vi "MethodGuide.vi"(1 "Attributes":string[](array[string])) -> (15 "Preview":string, 16 "Canceled":bool)   [LabVIEW 2020, in "DQMHModuleNode.lvclass"]
uses:
  <resource>/Framework/Providers/Open_GDS/UML/DQMHModuleNode_class/DQMHModuleNode.lvclass
  <resource>/Framework/Providers/Open_GDS/UML/DQMHModuleNode_class/EventType.ctl
  <resource>/Framework/Providers/Open_GDS/UML/ContextHelp/ContextHelp_HelpTexts.ctl
panel:
  in  "Roundtrip : Broadcast":string caption="Name of Roundtrip Broadcast"
  in  "Type":T1
  in  "Help":bool
  in  "Cancel":bool
  in  "OK":bool
  in  "Event Name":string(combo) caption="Name of Roundtrip Request"
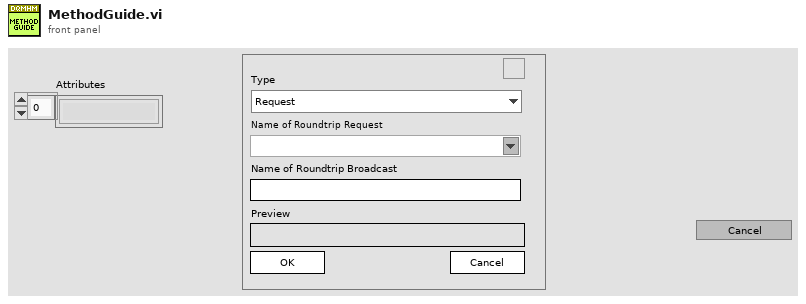
[diagram p1: front panel]
types:
  T1 = typedef "DQMHModuleNode.lvclass/EventType.ctl" = enum16{"Request", "Request and Wait For Reply", "Roundtrip", "Broadcast"}
  T2 = enum8{"Enabled", "Disabled", "Disabled and Grayed Out"}
  T3 = typedef "ContextHelp_HelpTexts.ctl" = enum16{"None(Hide)", "Default", "Help", "Welcome", "GettingStarted", "ClassDiagram_Help", "SequenceDiagram_Help", "UseCaseDiagram_Help", "BSelect", "BClass", "BInterface", "BPackage", "BNote", "BDependency", "BInheritance", "BInterfaceImplementation", "BAssociation", "BAggregation", "BCompAggregation", "BNoteConnector", "BObject", "BActionBar", "BCall", "BSystem", "BActor", "BUseCase", "BGeneralization", "BIncludes", "BExtends", "BUseCaseDiagramAssociation", "ClassRelationshipEdge editDialog_Bent Style", "ClassRelationshipEdge editDialog_RelationType", "ClassRelationshipEdge editDialog_Reverse association", "ClassRelationshipEdge editDialog_Start label", "ClassRelationshipEdge editDialog_Middle label", "ClassRelationshipEdge editDialog_End label", "UMLEditor reversedEngineering_Pathes", "ReversedEngineering StateReverseDialog_Help", "ReversedEngineering StateQueuedSettings_Help", "UMLEditor reversedEngineering_AddTopVIs", "UMLEditor reversedEngineering_AddClasses", "UMLEditor reversedEngineering_AddDirs", "UMLEditor reversedEngineering_Recursively", "UMLEditor reversedEngineering_Remove", "UMLEditor reversedEngineering_ClearList", "UMLEditor reversedEngineering_HideSubAss", "UMLEditor reversedEngineering_CreateTypes", "UMLEditor reversedEngineering_OnlyInheritance", "UMLEditor reversedEngineering_CreateApplication", "UMLEditor reversedEngineering_OK", "UMLEditor reversedEngineering_Cancel", "UMLEditor reversedEngineering_Help", "UMLEditor createWizardScriptFile_ScriptfilePath", "UMLEditor createWizardScriptFile_ClassPath", "UMLEditor createWizardScriptFile_Use", "UMLEditor createWizardScriptFile_PrivateDirName", "UMLEditor createWizardScriptFile_DirAppend", "UMLEditor createWizardScriptFile_Separator Character", "UMLEditor createWizardScriptFile_OK", "UMLEditor createWizardScriptFile_Cancel", "UMLEditor createWizardScriptFile_Help", "ClassNode editDialog_Class Name", "InterfaceNode editDialog_Class Name", "ClassNode editDialog_Attribute", "ClassNode editDialog_Methods", "InterfaceNode editDialog_Methods", "ClassNode editDialog_connection", "InterfaceNode editDialog_connection", "ClassNode editDialog_StereoType", "ClassNode editDialog_ShowAttrib", "ClassNode editDialog_ShowMethods", "ClassNode editDialog_ClassPath", "ClassNode editDialog_AddAttribute", "ClassNode editDialog_AddMethod", "InterfaceNode editDialog_AddMethod", "ClassNode AttributeGuide_AttributeName", "ClassNode AttributeGuide_Array?", "ClassNode AttributeGuide_Data Type", "ClassNode AttributeGuide_RefName", "ClassNode AttributeGuide_Preview", "ClassNode AttributeGuide_OK", "ClassNode AttributeGuide_Cancel", "ClassNode MethodGuide_Visibility", "ClassNode MethodGuide_Method Name", "ClassNode MethodGuide_Preview", "ClassNode MethodGuide_OK", "ClassNode MethodGuide_Cancel", "CallNode EditCallProperties_AllButtons", "ObjectNode EditObjectlProperties_AllButtons", "ActorNode EditActorProperties_AllButtons", "UseCaseRelationshipNode EditUseCaselProperties_AllButtons", "UseCaseNode EditUseCaselProperties_AllButtons", "SystemNode EditSystemProperties_AllButtons", "ReversedEngineering UpdateAttributes_AllButtons", "StateNode editDialog_AllButtons", "StateTransition editDialog_AllButtons", "ArrangeNodes Main_Picture", "ArrangeNodes Main_Zoom", "ArrangeNodes Main_Auto Zoom", "ArrangeNodes Main_shorten", "ArrangeNodes Main_Min Length", "ArrangeNodes Main_Max Length", "ArrangeNodes Main_increase", "ArrangeNodes Main_decrease", "ArrangeNodes Main_Shake", "ArrangeNodes Main", "BState", "BInitialState", "BFinalState", "BStateTransition", "StateDiagram_Help", "StateDiagram_PropertiesAllButtons", "ReversedEngineering StateReverseDialog_ClearStates", "ReversedEngineering StateReverseDialog_UseQueuedStateMachines", "ReversedEngineering StateReverseDialog_QueuedSettings", "ReversedEngineering StateReverseDialog_SearchForVIs", "ReversedEngineering StateReverseDialog_SearchCriteria", "OptionsDialog_ClassBasePath", "OptionsDialog_VIPath", "OptionsDialog_ApplicationPath", "OptionsDialog_WizDir", "OptionsDialog_IniFilePath", "OptionsDialog_DefineColors", "OptionsDialog_Help", "OptionsDialog_CreateTypes", "ClassRelationshipEdge editDialog_SplitWire"}
  T4 = typedef "ContextHelp_ShowType.ctl" = cluster{"Header":string, "Picture":picture, "Text":string}
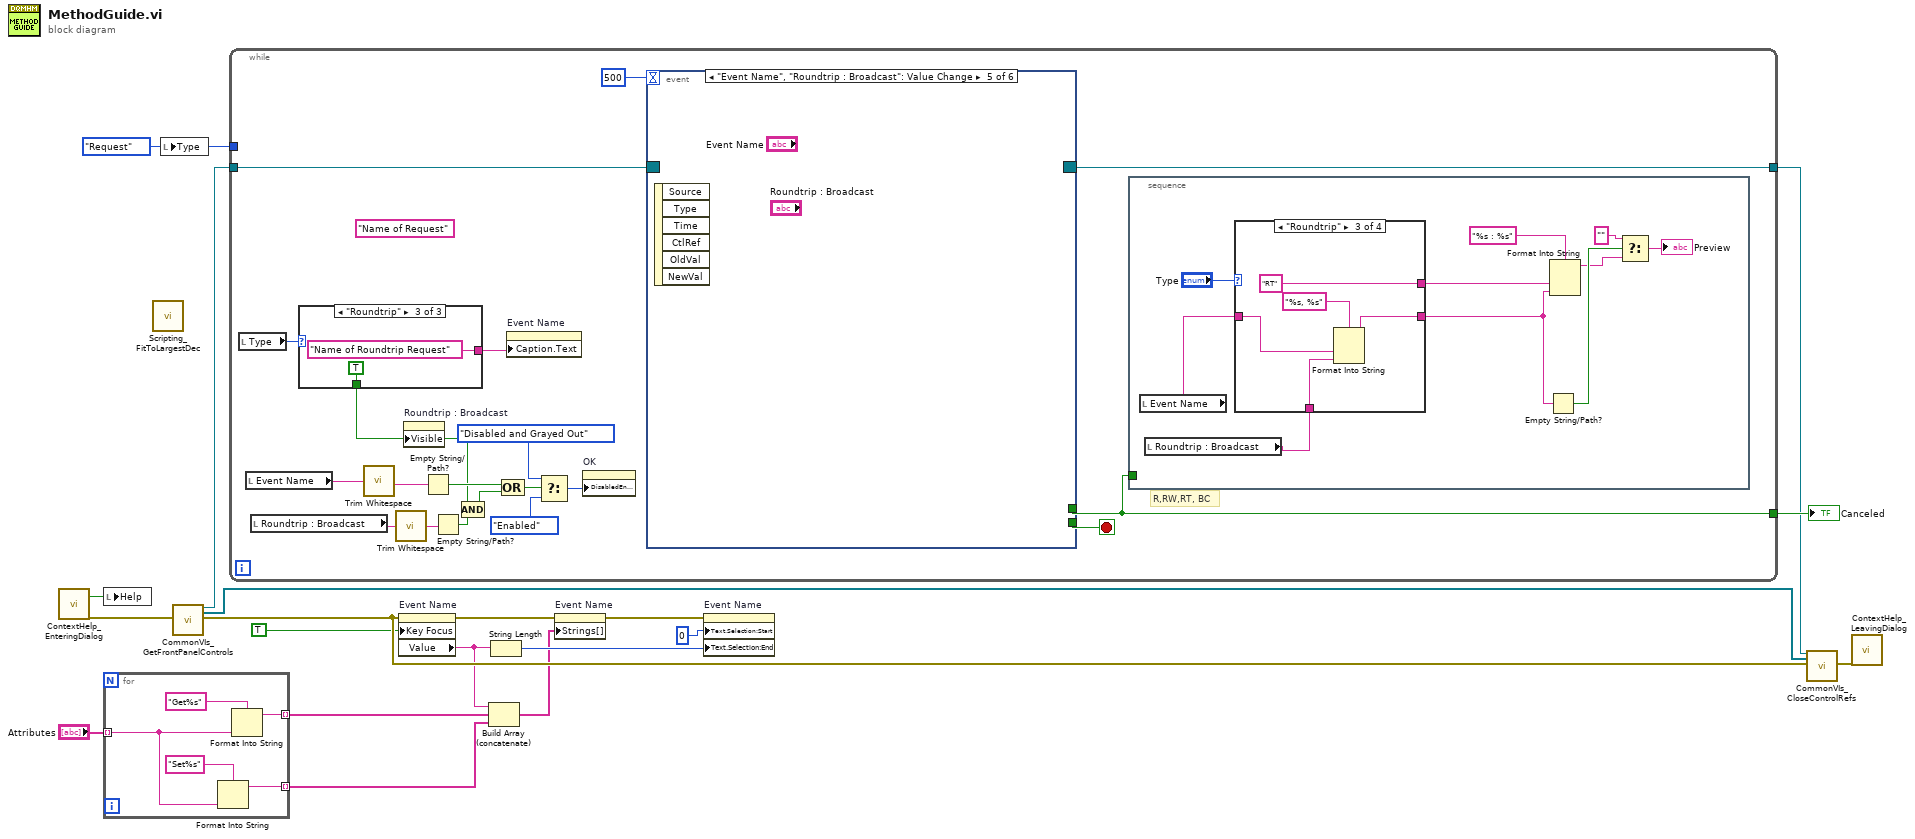
[diagram p0: block diagram]
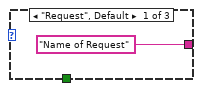
[diagram p2: hidden frame]
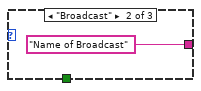
[diagram p3: hidden frame]
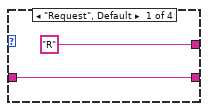
[diagram p4: hidden frame]
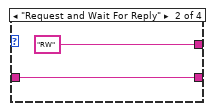
[diagram p5: hidden frame]
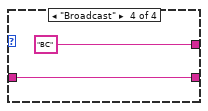
[diagram p6: hidden frame]
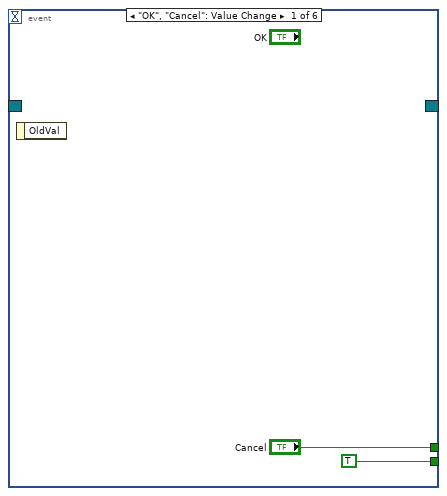
[diagram p7: hidden frame]
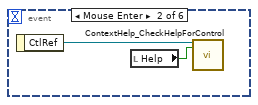
[diagram p8: hidden frame]
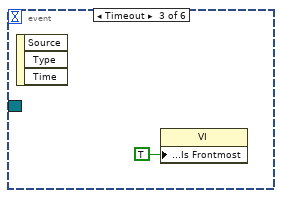
[diagram p9: hidden frame]
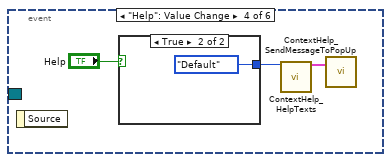
[diagram p10: hidden frame]
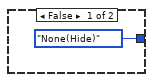
[diagram p11: hidden frame]
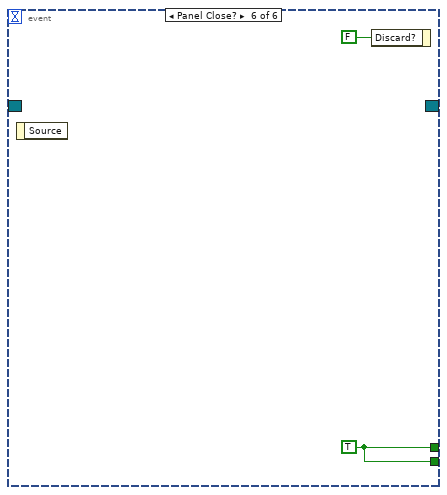
[diagram p12: hidden frame]
diagram:
  w1 = EventType."Request" ("Type")
  n1 = call <resource>:"ContextHelp_EnteringDialog.vi"() -> ("HelpStatus"=w18:bool, "error out"=w16:errorcluster)  [unwired: 3 in, 15 out]
  n2 = local write "Help"(w18) -> ()
  n3 = for {
    tunnel: [w21] -> w4 mode=indexing
    tunnel: "Attributes" -> [w22] mode=indexing
    tunnel: [w20] -> w2 mode=indexing
    n4 = Format Into String(format string="Set%s", w22) -> (resulting string=w20:string)  [unwired: 2 in, 1 out]
    n5 = Format Into String(format string="Get%s", w22) -> (resulting string=w21:string)  [unwired: 2 in, 1 out]
  }
  n6 = call <resource>:"Scripting_FitToLargestDec.vi"() -> ()  [unwired: 6 in, 2 out]
  n7 = local write "Type"(w1) -> ()
  n8 = call <resource>:"CommonVIs_GetFrontPanelControls.vi"("error in (no error)"=w16) -> ("Event Registration Refnum"=w14:refnum<event-registration>, "ControlRefs"=w17:refnum<vi>[], "error out"=w12:errorcluster)  [unwired: 1 in, 15 out]
  n9 = while {
    tunnel: [w39] -> w19
    tunnel: w14 -> [w42]
    tunnel: [w41] -> w13
    tunnel: w1 -> [_]
    stop <- w43 stop-if-true
    (unwired) "Name of Request" ("format string")
    # "R,RW,RT, BC"
    n10 = local read "Type"() -> (w38:T1)
    n11 = local read "Event Name"() -> (w36:string)
    n12 = local read "Roundtrip : Broadcast"() -> (w35:string)
    n13 = case shown="\"Roundtrip\"" w38 {
      tunnel: ["Name of Request" ("format string") "Name of Broadcast" ("format string") "Name of Roundtrip Request" ("format string")] -> w37
      tunnel: [_ _ TRUE] -> w26
      frame "Request", Default {
      }
      frame "Broadcast" {
      }
      frame "Roundtrip" {
      }
    }
    n14 = call <vilib>:"Trim Whitespace.vi"("string"=w36) -> ("trimmed string"=w34:string)  [unwired: 1 in]
    n15 = call <vilib>:"Trim Whitespace.vi"("string"=w35) -> ("trimmed string"=w28:string)  [unwired: 1 in]
    n16 = property on="Roundtrip : Broadcast" class="Str"("Visible"=w26) -> ()  [unwired: 2 in, 2 out]
    n17 = Empty String/Path?(string/path=w34) -> (empty?=w33:bool)
    n18 = Empty String/Path?(string/path=w28) -> (empty?=w27:bool)
    n19 = Compound Arithmetic op=AND(w26, w27) -> (w25:bool)
    n20 = Compound Arithmetic op=OR(w33, w25) -> (w32:bool)
    n21 = property on="Event Name" class="CmbBox"("Caption.Text"=w37) -> ()  [unwired: 2 in, 2 out]
    n22 = Select(t=T2."Disabled and Grayed Out" ("Disabled"), s=w32, f=T2."Enabled" ("Disabled")) -> (s? t:f=w31:T2)
    n23 = property on="OK" class="Bool"("DisabledEnum"=w31) -> ()  [unwired: 2 in, 2 out]
    n24 = event shown="[4] \"Event Name\", \"Roundtrip : Broadcast\": Value Change" {
      selector: w42 -> [_ _ _ _ _ _]
      dyn-events: [_ _ _ _ _ _] -> w41
      timeout: 500 -> [_ _ _ _ _ _]
      tunnel: ["Cancel" _ _ _ _ w79] -> w39
      tunnel: [TRUE _ _ _ _ w79] -> w43
      event "OK", "Cancel": Value Change {
        n25 = event-data() -> ()  [unwired: 2 out]
      }
      event Mouse Enter {
        n26 = event-data() -> ("CtlRef"=w71:refnum<vi>)  [unwired: 1 out]
        n27 = local read "Help"() -> (w72:bool)
        n28 = call <resource>:"ContextHelp_CheckHelpForControl.vi"("Ctl Refnum"=w71, "Help"=w72) -> ()  [unwired: 1 in, 17 out]
      }
      event Timeout {
        n29 = event-data() -> ()  [unwired: 4 out]
        n30 = property class="VI"("Front Panel Window:Is Frontmost"=TRUE) -> ()  [unwired: 2 in, 2 out]
      }
      event "Help": Value Change {
        n31 = event-data() -> ()  [unwired: 2 out]
        n32 = case shown="True" "Help" {
          tunnel: [ContextHelp_HelpTexts."None(Hide)" ("HelpText") ContextHelp_HelpTexts."Default" ("HelpText")] -> w75
          frame False {
          }
          frame True {
          }
        }
        n33 = call <resource>:"ContextHelp_HelpTexts.vi"("HelpText (enum or string)"=w75) -> ("HelpOut"=w76:T4)  [unwired: 18 out]
        n34 = call <resource>:"ContextHelp_SendMessageToPopUp.vi"("PopUpMessage"=w76) -> ()  [unwired: 2 in, 17 out]
      }
      event "Event Name", "Roundtrip : Broadcast": Value Change {
        n35 = event-data() -> ()  [unwired: 7 out]
      }
      event Panel Close? {
        w79 = TRUE ("Discard?")
        n36 = event-data() -> ()  [unwired: 2 out]
        n37 = event-data("Discard?"=FALSE) -> ()  [unwired: 1 in, 1 out]
      }
    }
    n38 = stacked-sequence {
      tunnel: w39 -> [_]
      frame #0 {
        n39 = local read "Event Name"() -> (w50:string)
        n40 = local read "Roundtrip : Broadcast"() -> (w48:string)
        n41 = case shown="\"Roundtrip\"" "Type" {
          tunnel: ["R" "RW" "RT" "BC"] -> w51
          tunnel: w50 -> [w58 w60 w64 w67]
          tunnel: [w58 w60 w62 w67] -> w49
          tunnel: w48 -> [_ _ w63 _]
          frame "Request", Default {
          }
          frame "Request and Wait For Reply" {
          }
          frame "Roundtrip" {
            n42 = Format Into String(format string="%s, %s", w64, w63) -> (resulting string=w62:string)  [unwired: 2 in, 1 out]
          }
          frame "Broadcast" {
          }
        }
        n43 = Empty String/Path?(string/path=w49) -> (empty?=w56:bool)
        n44 = Format Into String(format string="%s : %s", w51, w49) -> (resulting string=w55:string)  [unwired: 2 in, 1 out]
        n45 = Select(t="", s=w56, f=w55) -> (s? t:f=→"Preview":string)
      }
    }
  }
  "Canceled" <- w19
  n46 = property on="Event Name" class="CmbBox"(error in=w12, "Key Focus"=TRUE ("Front Panel Window:Is Frontmost")) -> (error out=w8:errorcluster, "Value"=w6:string)  [unwired: 1 in, 1 out]
  n47 = Build Array (concatenate)(w6, w4, w2) -> (w5:string[])
  n48 = String Length(string=w6) -> (length=w9:i32)
  n49 = property on="Event Name" class="CmbBox"(error in=w8, "Strings[]"=w5) -> (error out=w7:errorcluster)  [unwired: 1 in, 1 out]
  n50 = property on="Event Name" class="CmbBox"(error in=w7, "Text.Selection:Start"=u32 0, "Text.Selection:End"=w9) -> ()  [unwired: 1 in, 2 out]
  n51 = call <resource>:"CommonVIs_CloseControlRefs.vi"("Event Registration Refnum"=w13, "ControlRefs"=w17, "error in (no error)"=w12) -> ("error out"=w15:errorcluster)  [unwired: 16 out]
  n52 = call <resource>:"ContextHelp_LeavingDialog.vi"("error in (no error)"=w15) -> ()  [unwired: 2 in, 17 out]
